vi "Set Sampling Interval.vi"(8 "error in (no error)":errorcluster, 9 "Sampling Interval (s)":u32=1, 11 "EPU452 in":refnum<class "EPU452.lvclass">) -> (0 "error out":errorcluster, 2 "Response":string, 3 "EPU452 out":refnum<class "EPU452.lvclass">)   [LabVIEW 2018, in "EPU452.lvclass"]
uses:
  EPU452.lvclass
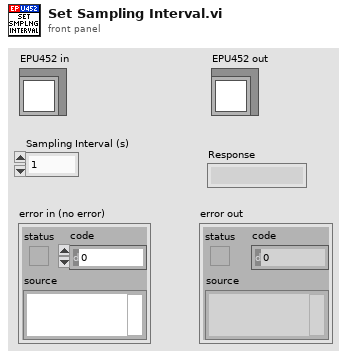
[diagram p1: front panel]
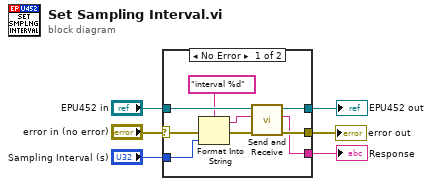
[diagram p0: block diagram]
diagram:
  n1 = case shown="No Error" "error in (no error)" {
    selector: "error in (no error)" -> [w12 w17]
    tunnel: [w9 w17] -> w5
    tunnel: [w8 w16] -> w3
    tunnel: "EPU452 in" -> [w15 w16]
    tunnel: "Sampling Interval (s)" -> [w11 _]
    tunnel: [w7 _] -> w1
    frame No Error {
      n2 = Format Into String(format string="interval %d", error in=w12, w11) -> (resulting string=w13:string, error out=w14:errorcluster)  [unwired: 1 in]
      n3 = call "Send and Receive.vi"("error in (no error)"=w14, "Command"=w13, "EPU452 in"=w15) -> ("error out"=w9:errorcluster, "Response"=w7:string, "EPU452 out"=w8:refnum<class "EPU452.lvclass">)  [unwired: 6 in]
    }
    frame Error {
    }
  }
  "error out" <- w5
  "EPU452 out" <- w3
  "Response" <- w1
